vi "Test.vi"() -> ()   [LabVIEW 2022 SP3, in "TcpServer.lvlib"]
uses:
  TcpServer.lvlib
  TcpServer/TcpServer.lvclass
  C:/Program Files (x86)/National Instruments/LabVIEW 2022/vi.lib/ActorFramework/Actor/Actor.lvclass
  <vilib>/ActorFramework/Reply Msg/Reply Msg.lvclass/Reply Msg.ctl
  <vilib>/ActorFramework/Message Enqueuer/Message Enqueuer.lvclass/Message Enqueuer.ctl
  <vilib>/ActorFramework/Report Error Msg/Report Error Msg.lvclass/Report Error Msg.ctl
  DataReceived/DataReceived.lvclass/DataReceived.ctl
  ServerConfig/ServerConfig.lvclass
  ServerConfig/ServerConfig.lvclass/ServerConfig.ctl
  TcpServer Messages/ServerConfig Msg/ServerConfig Msg.lvclass/ServerConfig Msg.ctl
  DataReceived/Read TimeStamp.vi
  DataReceived/Read Refnum.vi
  DataReceived/Read Data.vi
  ServerConfig/Write Address.vi
  ServerConfig/Write Port.vi
  ServerConfig/Write ReadMode.vi
  ServerConfig/Write OpenTimeout.vi
  ServerConfig/Write ReadTimeout.vi
  ServerConfig/Write WriteTimeout.vi
  ServerConfig/Write ConnectionTimeout.vi
  ServerConfig/Write MaxNumberOfConnections.vi
  ServerConfig/Write ConnectionLifetime.vi
  ServerConfig/Write WaitForConnectionDelay.vi
  ServerConfig/Write ReceiveDataBufferSize.vi
  <vilib>/ActorFramework/Reply Msg/Send Message And Wait For Response.vi
  <vilib>/ActorFramework/Message Enqueuer/Enqueue.vi
  TcpServer Messages/GetReceiveDataBuffer Msg/GetReceiveDataBuffer Msg.lvclass
  C:/Program Files (x86)/National Instruments/LabVIEW 2022/vi.lib/ActorFramework/Reply Msg/Reply Msg.lvclass
  <vilib>/ActorFramework/Reply Msg/Reply Msg.lvclass
  C:/Program Files (x86)/National Instruments/LabVIEW 2022/vi.lib/ActorFramework/Message/Message.lvclass
  <vilib>/ActorFramework/Report Error Msg/Report Error Msg.lvclass
  TcpServer Messages/ServerConfig Msg/ServerConfig Msg.lvclass
  TcpServer Messages/ServerStart Msg/ServerStart Msg.lvclass
  TcpServer Messages/ServerStop Msg/ServerStop Msg.lvclass
  <vilib>/ActorFramework/Stop Msg/Stop Msg.lvclass
  <vilib>/ActorFramework/Message Priority Queue/Priority Enqueue.vi
  DataReceived/DataReceived.lvclass
  <vilib>/ActorFramework/Actor/Actor.lvclass
panel:
  out "# elements in queue":i32
  out "Time":string
  out "Data":string
  out "Refnum":u64
  in  "Server Config":T1={"Address"="127.0.0.1", "Port"=0, "ReadMode"=enum."Standard", "OpenTimeout"=5000, "ReadTimeout"=5000, "WriteTimeout"=5000, "ConnectionTimeout"=5000, "MaxNumberOfConnections"=5, "ConnectionLifetime"=5000, "WaitForConnectionDelay"=1000, "ReceiveDataBufferSize"=1000}
  in  "BtnServerStop":bool
  in  "BtnServerStart":bool
  out "error out":errorcluster
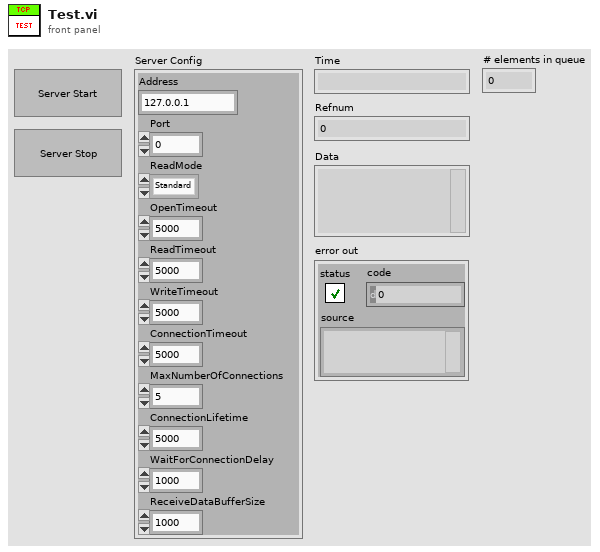
[diagram p1: front panel]
types:
  T1 = cluster{"Address":string, "Port":u16, "ReadMode":enum16{"Standard", "Buffered", "CRLF", "Immediate"}, "OpenTimeout":i32, "ReadTimeout":i32, "WriteTimeout":i32, "ConnectionTimeout":i32, "MaxNumberOfConnections":i32, "ConnectionLifetime":i32, "WaitForConnectionDelay":i32, "ReceiveDataBufferSize":i32}
  T2 = enum16{"Standard", "Buffered", "CRLF", "Immediate"}
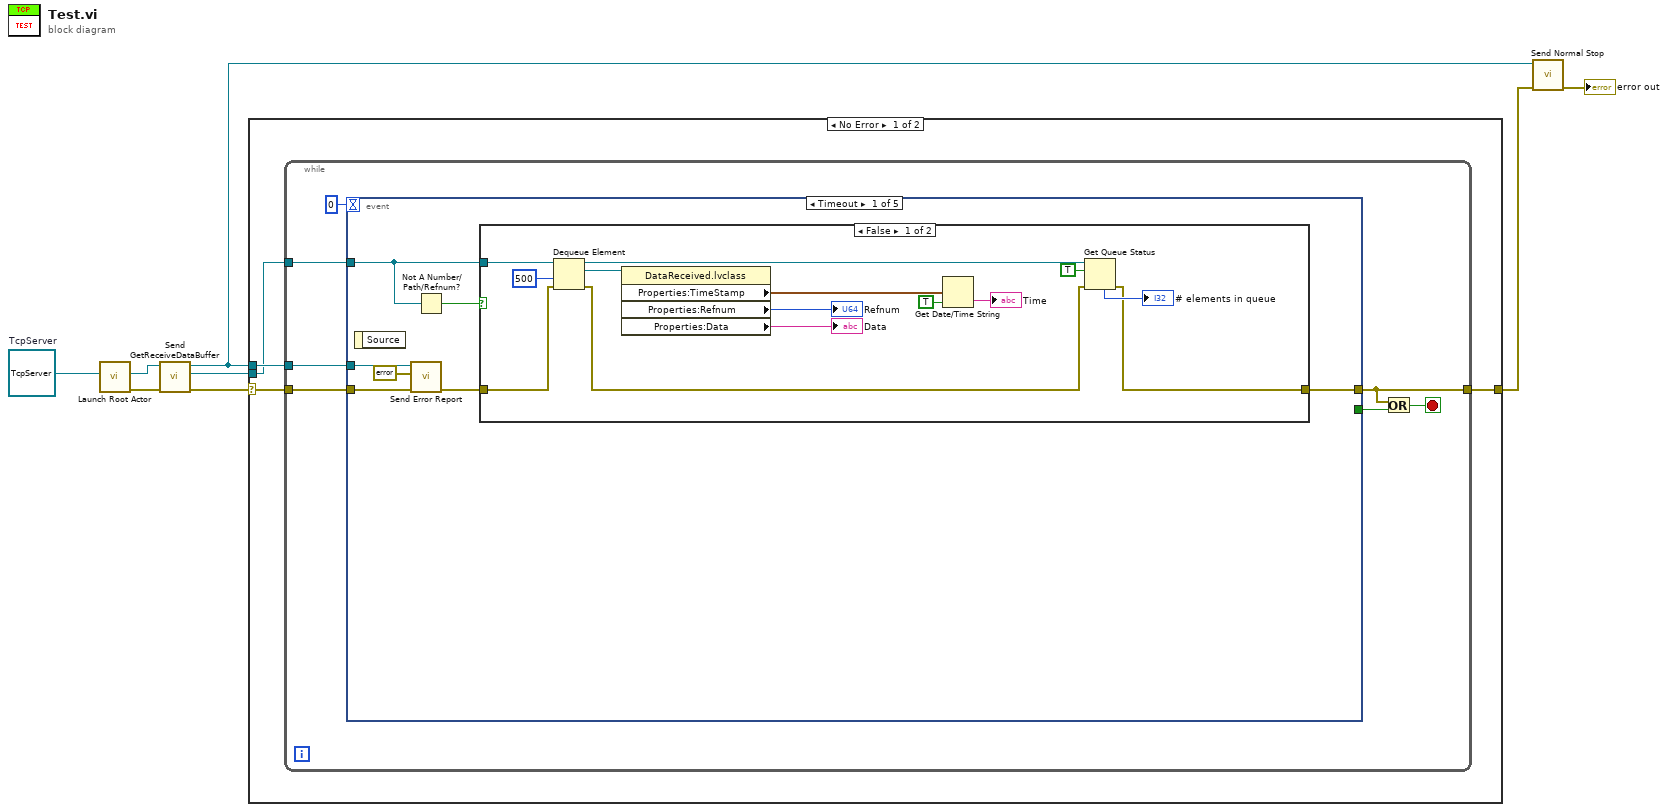
[diagram p0: block diagram]
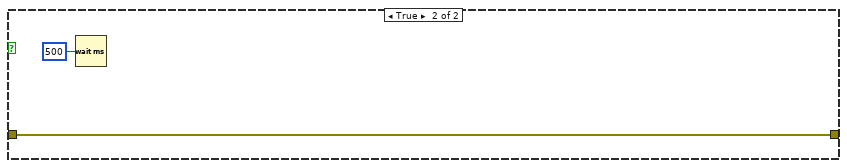
[diagram p2: hidden frame]
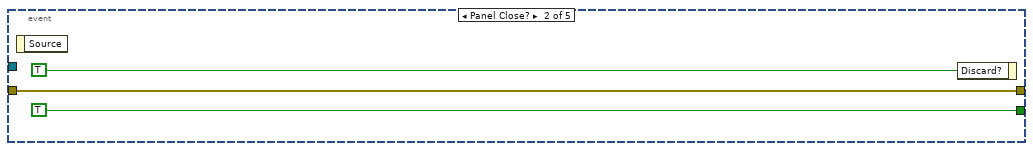
[diagram p3: hidden frame]
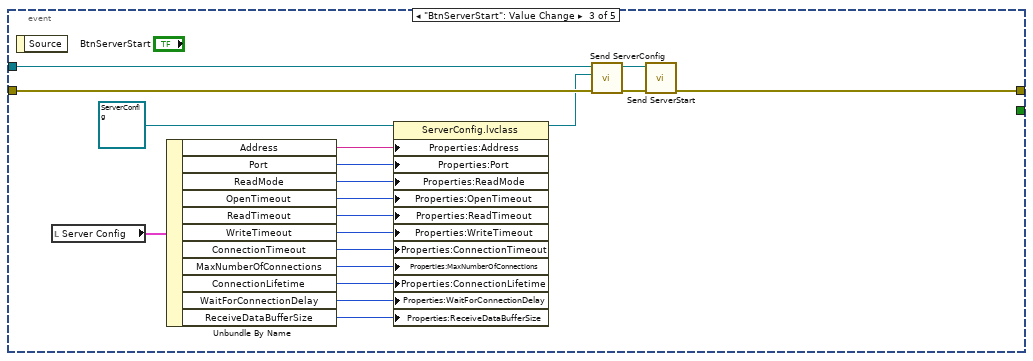
[diagram p4: hidden frame]
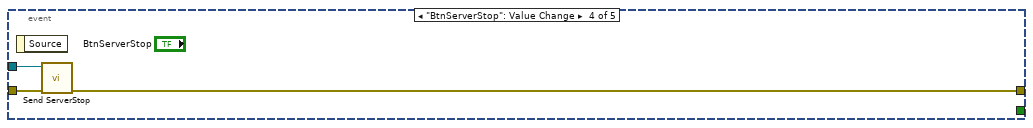
[diagram p5: hidden frame]
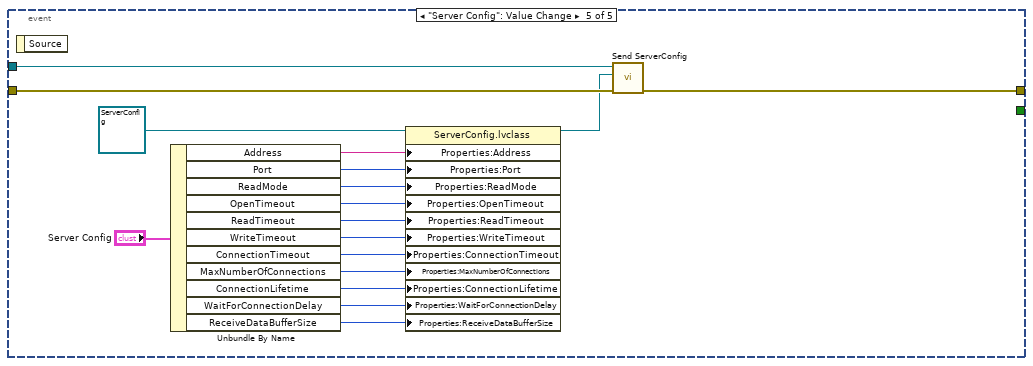
[diagram p6: hidden frame]
diagram:
  w8 = refnum<class "TcpServer.lvclass"> refnum  # TcpServer
  n1 = call <vilib>:"Launch Root Actor.vi"("Actor"=w8) -> ("error out"=w1:errorcluster, "Actor's Enqueuer"=w5:refnum<class "Message Enqueuer.lvclass">)  [unwired: 9 in]
  n2 = call "Send GetReceiveDataBuffer.vi"("error in (no error)"=w1, "Message Enqueuer"=w5) -> ("error out"=w3:errorcluster, "ReceiveDataBuffer"=w2:refnum<queue>, "Message Enqueuer out"=w4:refnum<class "Message Enqueuer.lvclass">)  [unwired: 6 in, 1 out]
  n3 = case shown="No Error" w3 {
    selector: w3 -> [w12 w85]
    tunnel: w4 -> [w11 _]
    tunnel: [w10 w85] -> w7
    tunnel: w2 -> [w9 _]
    frame No Error {
      n4 = while {
        tunnel: w11 -> [w18]
        tunnel: w12 -> [w19]
        tunnel: [w14] -> w10
        tunnel: w9 -> [w13]
        stop <- w16 stop-if-true
        n5 = event shown="[0] Timeout" {
          selector: _ -> [_ _ _ _ _]
          dyn-events: _ -> [_ _ _ _ _]
          timeout: 0 -> [_ _ _ _ _]
          tunnel: [_ TRUE ("Discard?") _ _ _] -> w15
          tunnel: w19 -> [w26 w44 w64 w66 w84]
          tunnel: [w22 w44 w52 w65 w82] -> w14
          tunnel: w18 -> [w25 _ w62 w67 w83]
          tunnel: w13 -> [w20 _ _ _ _]
          event Timeout {
            n6 = event-data() -> ()  [unwired: 1 in, 1 out]
            n7 = call <vilib>:"Send Error Report.vi"("error in (no error)"=w26, "Error From Sender"=errorcluster {"status"=FALSE, "code"=0, "source"=""}, "Message Enqueuer"=w25) -> ("error out"=w21:errorcluster)  [unwired: 8 in]
            n8 = Not A Number/Path/Refnum?(number/path/refnum=w20) -> (NaN/Path/Refnum?=w23:bool)
            n9 = case shown="False" w23 {
              tunnel: [w28 w42] -> w22
              tunnel: w21 -> [w38 w42]
              tunnel: w20 -> [w40 _]
              frame False {
                n10 = Dequeue Element(queue=w40, timeout in ms (-1)=500, error in (no error)=w38) -> (queue out=w39:refnum<queue>, element=w36:refnum<class "DataReceived.lvclass">, error out=w29:errorcluster)  [unwired: 1 out]
                n11 = property class="DataReceived.lvclass"(reference=w36) -> ("Properties:TimeStamp"=w33:timestamp, "Properties:Refnum"=→"Refnum":u64, "Properties:Data"=→"Data":string)  [unwired: 1 in, 2 out]
                n12 = Get Date/Time String(seconds (now)=w33, want seconds? (F)=TRUE) -> (time string=→"Time":string)  [unwired: 1 in, 1 out]
                n13 = Get Queue Status(queue=w39, return elements? (F)=TRUE, error in (no error)=w29) -> (error out=w28:errorcluster, # elements in queue=→"# elements in queue":i32)  [unwired: 6 out]
              }
              frame True {
                n14 = Wait (ms)(milliseconds to wait=u32 500) -> ()  [unwired: 1 out]
              }
            }
          }
          event Panel Close? {
            n15 = event-data() -> ()  [unwired: 1 in, 1 out]
            n16 = event-data("Discard?"=TRUE) -> ()  [unwired: 1 in, 1 out]
          }
          event "BtnServerStart": Value Change {
            n17 = event-data() -> ()  [unwired: 1 in, 1 out]
            n18 = local read "Server Config"() -> (w55:T1)
            n19 = Unbundle By Name(w55) -> ("Address"=w51:string, "Port"=w50:u16, "ReadMode"=w59:T2, "OpenTimeout"=w58:i32, "ReadTimeout"=w57:i32, "WriteTimeout"=w56:i32, "ConnectionTimeout"=w53:i32, "MaxNumberOfConnections"=w49:i32, "ConnectionLifetime"=w48:i32, "WaitForConnectionDelay"=w47:i32, "ReceiveDataBufferSize"=w46:i32)
            n20 = property class="ServerConfig.lvclass"(reference=refnum<class "ServerConfig.lvclass"> refnum ("ServerConfig"), "Properties:Address"=w51, "Properties:Port"=w50, "Properties:ReadMode"=w59, "Properties:OpenTimeout"=w58, "Properties:ReadTimeout"=w57, "Properties:WriteTimeout"=w56, "Properties:ConnectionTimeout"=w53, "Properties:MaxNumberOfConnections"=w49, "Properties:ConnectionLifetime"=w48, "Properties:WaitForConnectionDelay"=w47, "Properties:ReceiveDataBufferSize"=w46) -> (reference out=w54:refnum<class "ServerConfig.lvclass">)  [unwired: 1 in, 1 out]
            n21 = call "Send ServerConfig.vi"("error in (no error)"=w64, "ServerConfig"=w54, "Message Enqueuer"=w62) -> ("error out"=w63:errorcluster, "Message Enqueuer out"=w61:refnum<class "Message Enqueuer.lvclass">)  [unwired: 7 in]
            n22 = call "Send ServerStart.vi"("error in (no error)"=w63, "Message Enqueuer"=w61) -> ("error out"=w52:errorcluster)  [unwired: 8 in, 1 out]
          }
          event "BtnServerStop": Value Change {
            n23 = event-data() -> ()  [unwired: 1 in, 1 out]
            n24 = call "Send ServerStop.vi"("error in (no error)"=w66, "Message Enqueuer"=w67) -> ("error out"=w65:errorcluster)  [unwired: 8 in, 1 out]
          }
          event "Server Config": Value Change {
            n25 = event-data() -> ()  [unwired: 1 in, 1 out]
            n26 = Unbundle By Name("Server Config") -> ("Address"=w73:string, "Port"=w72:u16, "ReadMode"=w78:T2, "OpenTimeout"=w77:i32, "ReadTimeout"=w76:i32, "WriteTimeout"=w75:i32, "ConnectionTimeout"=w74:i32, "MaxNumberOfConnections"=w71:i32, "ConnectionLifetime"=w70:i32, "WaitForConnectionDelay"=w69:i32, "ReceiveDataBufferSize"=w68:i32)
            n27 = property class="ServerConfig.lvclass"(reference=refnum<class "ServerConfig.lvclass"> refnum ("ServerConfig"), "Properties:Address"=w73, "Properties:Port"=w72, "Properties:ReadMode"=w78, "Properties:OpenTimeout"=w77, "Properties:ReadTimeout"=w76, "Properties:WriteTimeout"=w75, "Properties:ConnectionTimeout"=w74, "Properties:MaxNumberOfConnections"=w71, "Properties:ConnectionLifetime"=w70, "Properties:WaitForConnectionDelay"=w69, "Properties:ReceiveDataBufferSize"=w68) -> (reference out=w80:refnum<class "ServerConfig.lvclass">)  [unwired: 1 in, 1 out]
            n28 = call "Send ServerConfig.vi"("error in (no error)"=w84, "ServerConfig"=w80, "Message Enqueuer"=w83) -> ("error out"=w82:errorcluster)  [unwired: 7 in, 1 out]
          }
        }
        n29 = Or(x=w14, y=w15) -> (x .or. y?=w16:bool)
      }
    }
    frame Error {
    }
  }
  n30 = call <vilib>:"Send Normal Stop.vi"("error in (no error)"=w7, "Message Enqueuer"=w4) -> ("error out"=→"error out":errorcluster)  [unwired: 9 in]
